vi "Q -- range -- not.vi"(1 "new state":T1=enum."above") -> (0 "new state out":T1)   [LabVIEW 2010]
uses:
  comparison control.ctl
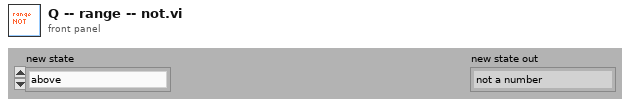
[diagram p1: front panel]
types:
  T1 = typedef "comparison control.ctl" = enum16{"not a number", "above", "in range", "below"}
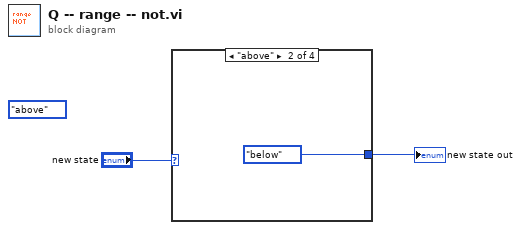
[diagram p0: block diagram]
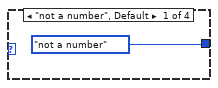
[diagram p2: hidden frame]
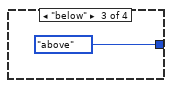
[diagram p3: hidden frame]
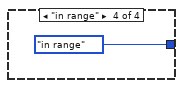
[diagram p4: hidden frame]
diagram:
  (unwired) comparison_control."above" ("new state")
  n1 = case shown="\"above\"" "new state" {
    tunnel: [comparison_control."not a number" ("new state") comparison_control."below" ("new state") comparison_control."above" ("new state") comparison_control."in range" ("new state")] -> w1
    frame "not a number", Default {
    }
    frame "above" {
    }
    frame "below" {
    }
    frame "in range" {
    }
  }
  "new state out" <- w1
